vi "Get Value.vi"(8 "error in (no error)":errorcluster, 11 "SingleB in":refnum<class "SingleB.lvclass">) -> (0 "error out":errorcluster, 2 "value":string, 3 "SingleB out":refnum<class "SingleB.lvclass">)   [LabVIEW 2020, in "SingleB.lvclass"]
uses:
  SingleB.lvclass
  D:/03 GitHub/LabVIEW-Singleton/Singleton/Singleton.lvclass
  Singleton/Singleton.lvclass/Singleton.ctl
  SingleB.lvclass/SingleB.ctl
  Singleton/Singleton.lvclass
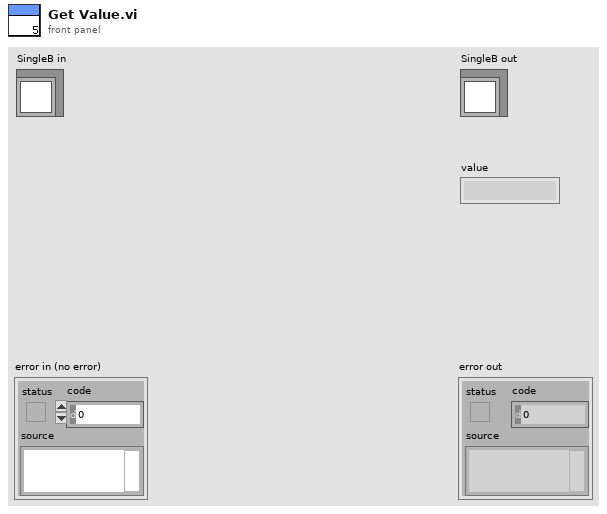
[diagram p1: front panel]
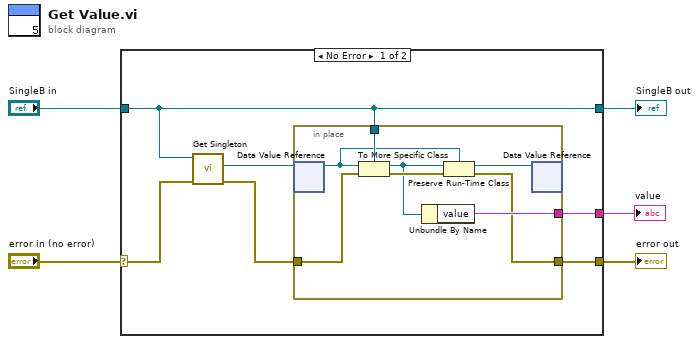
[diagram p0: block diagram]
diagram:
  n1 = case shown="No Error" "error in (no error)" {
    selector: "error in (no error)" -> [w8 w21]
    tunnel: [w7 w21] -> w3
    tunnel: [w10 w20] -> w2
    tunnel: "SingleB in" -> [w10 w20]
    tunnel: [w9 _] -> w1
    frame No Error {
      n2 = call "Get Singleton.vi"("error in (no error)"=w8, "Singleton in"=w10) -> ("error out"=w6:errorcluster, "singleton"=w11:refnum<data-value>)  [unwired: 7 in, 1 out]
      n3 = in-place {
        in-place-border: w10 -> [w19]
        in-place-border: [w18] -> w9
        in-place-border: w6 -> [w17]
        in-place-border: [w15] -> w7
        n4 = in-place-dvr #1(w11) -> (w14:refnum<class>)  [unwired: 1 out]
        n5 = To More Specific Class(target class=w19, reference=w14, error in=w17) -> (specific class reference=w13:refnum<class "SingleB.lvclass">, error out=w16:errorcluster)
        n6 = Unbundle By Name(w13) -> ("value"=w18:string)
        n7 = Preserve Run-Time Class(object in=w13, error in=w16, 2:w14) -> (object out=w12:refnum<class>, error out=w15:errorcluster)
        n8 = in-place-dvr #1(w12) -> ()  [unwired: 2 out]
      }
    }
    frame Error {
    }
  }
  "error out" <- w3
  "SingleB out" <- w2
  "value" <- w1
